vi "WS1050 CAPDAC Setting.vi"(8 "error in":errorcluster, 11 "Write Reg I2C":u8=11 caption="Register" format="0x%02x") -> (0 "error out":errorcluster, 3 "AD7747 Values":string[][](table))   [LabVIEW 2012]
uses:
  Type Defs/WSVCAP SHL I2C DUT Mask Mode Enum.ctl
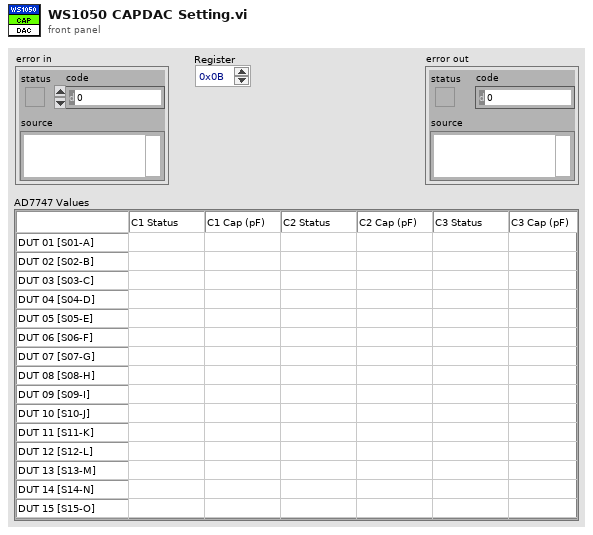
[diagram p1: front panel]
types:
  T1 = typedef "WSVCAP SHL I2C DUT Mask Mode Enum.ctl" = enum16{"Custom", "C1", "C2", "C3", "All"}
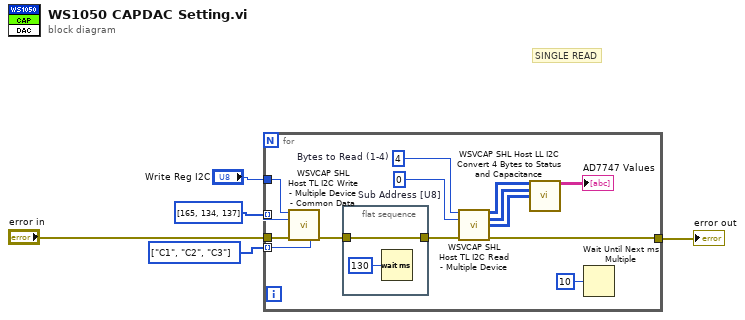
[diagram p0: block diagram]
diagram:
  w1 = T1[] [enum."C1", enum."C2", enum."C3"] items=["Custom", "C1", "C2", "C3", "All"]
  # "SINGLE READ"
  n1 = for {
    tunnel: "error in" -> [w19]
    tunnel: u8[] [165, 134, 137] -> [w18] mode=indexing
    tunnel: [w8] -> w3
    tunnel: "Write Reg I2C" -> [w7]
    tunnel: w1 -> [w6] mode=indexing
    w11 = u8 4  # Bytes to Read (1-4)
    w10 = u8 0  # Sub Address [U8]
    n2 = call "WSVCAP SHL Host TL I2C Write - Multiple Device - Common Data.vi"("Sub Address"=w7, "Data Out [U8]"=w18, "error in"=w19, "DUT Mask Mode (All)"=w6) -> ("error out"=w9:errorcluster)  [unwired: 11 in]
    n3 = flat-sequence {
      tunnel: w9 -> [w20]
      tunnel: [w20] -> w16
      frame #0 {
        n4 = Wait (ms)(milliseconds to wait=u32 130) -> ()  [unwired: 1 out]
      }
    }
    n5 = call "WSVCAP SHL Host TL I2C Read - Multiple Device.vi"("Bytes to Read (1-4)"=w11, "Sub Address [U8]"=w10, "error in"=w16) -> ("C1:1-16 Read Data [U8]"=w12:u8[][], "C2:1-16 Read Data [U8]"=w13:u8[][], "C3:1-16 Read Data [U8]"=w15:u8[][], "error out"=w8:errorcluster)  [unwired: 9 in]
    n6 = call "WSVCAP SHL Host LL I2C Convert 4 Bytes to Status and Capacitance.vi"("C1:1-16 Read Data [U8]"=w12, "C2_1-16 Read Data [U8]"=w13, "C3_1-16 Read Data [U8]"=w15) -> ("AD7747 Values"=→"AD7747 Values":string[][])  [unwired: 12 in]
    n7 = Wait Until Next ms Multiple(millisecond multiple=u32 10) -> ()  [unwired: 1 out]
  }
  "error out" <- w3
